vi "Replace All GUIDs.vi"(8 "error in":errorcluster, 10 "xml path":path, 11 "constants vi path":path) -> (0 "error out":errorcluster)   [LabVIEW 2020, in "Utility.lvlib"]
uses:
  Utility.lvlib
  NationalInstruments.VeriStand.XMLReader
  44b35cc9-1a06-4614-a9e3-699a5a99c799.vi
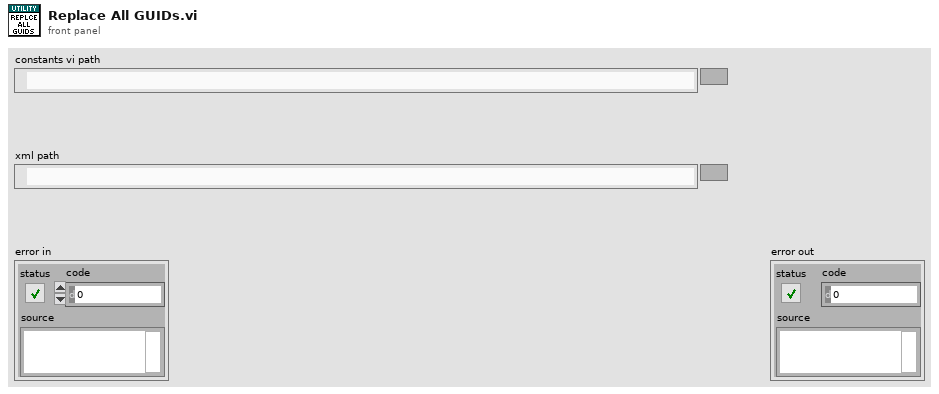
[diagram p1: front panel]
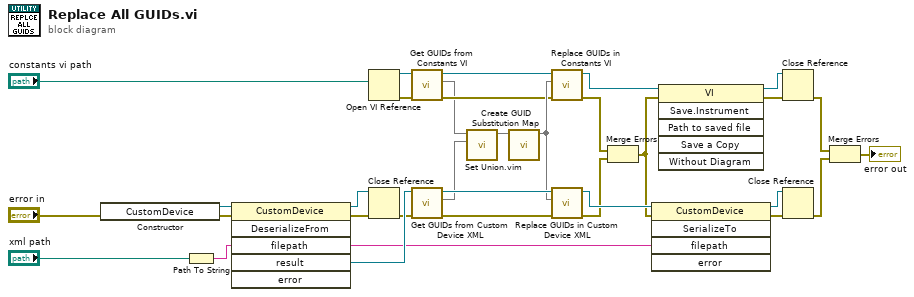
[diagram p0: block diagram]
diagram:
  n1 = constructor class="CustomDevice"(error in="error in") -> (reference out=w29:refnum<k24>, error out=w30:errorcluster)  [unwired: 2 in, 1 out]
  n2 = Path To String(path="xml path") -> (string=w21:string)
  n3 = invoke class="CustomDevice" method="DeserializeFrom"(reference=w29, error in=w30, "filepath"=w21) -> (reference out=w22:refnum<k24>, error out=w23:errorcluster, "result"=w27:refnum<k24>)  [unwired: 3 in, 3 out]
  n4 = Open VI Reference(vi path="constants vi path") -> (vi reference=w31:refnum<vi>, error out=w10:errorcluster)  [unwired: 5 in]
  n5 = Close Reference(reference=w22, error in (no error)=w23) -> (error out=w11:errorcluster)
  n6 = call "Get GUIDs from Constants VI.vi"("error in"=w10, "VI in"=w31) -> ("error out"=w12:errorcluster, "set out"=w9:set{string}, "VI out"=w18:refnum<vi>)  [unwired: 7 in]
  n7 = call "Get GUIDs from Custom Device XML.vi"("error in"=w11, "CustomDevice in"=w27) -> ("error out"=w13:errorcluster, "set out"=w8:set{string}, "CustomDevice out"=w25:refnum<k24>)  [unwired: 6 in]
  n8 = call "Set Union.vim"("set 2"=w8, "set 1"=w9) -> ("union"=w26:set{string})  [unwired: 9 in]
  n9 = call "Create GUID Substitution Map.vi"("guids"=w26) -> ("guid map"=w17:map{string, string})  [unwired: 10 in]
  n10 = call "Replace GUIDs in Constants VI.vi"("error in"=w12, "guid map"=w17, "VI in"=w18) -> ("error out"=w6:errorcluster, "VI out"=w16:refnum<vi>)  [unwired: 7 in]
  n11 = call "Replace GUIDs in Custom Device XML.vi"("error in"=w13, "guid map"=w17, "CustomDevice in"=w25) -> ("error out"=w7:errorcluster, "CustomDevice out"=w24:refnum<k24>)  [unwired: 6 in]
  n12 = Merge Errors(w6, w7) -> (w5:errorcluster)
  n13 = invoke class="CustomDevice" method="SerializeTo"(reference=w24, error in=w5, "filepath"=w21) -> (reference out=w19:refnum<k24>, error out=w20:errorcluster)  [unwired: 2 in, 3 out]
  n14 = invoke class="VI" method="Save.Instrument"(reference=w16, error in=w5) -> (reference out=w14:refnum<vi>, error out=w15:errorcluster)  [unwired: 4 in, 4 out]
  n15 = Close Reference(reference=w14, error in (no error)=w15) -> (error out=w4:errorcluster)
  n16 = Close Reference(reference=w19, error in (no error)=w20) -> (error out=w3:errorcluster)
  n17 = Merge Errors(w4, w3) -> (→"error out":errorcluster)
